vi "XImc example calb corr.vi"() -> ()   [LabVIEW 2012]
uses:
  libximc.lvlib
panel:
  in  "Correction table file.":path
  out "function return":i32
  out "Corrected position  Position":dbl
  out "Unrecorded position.":dbl
  in  "error in (no error)":errorcluster
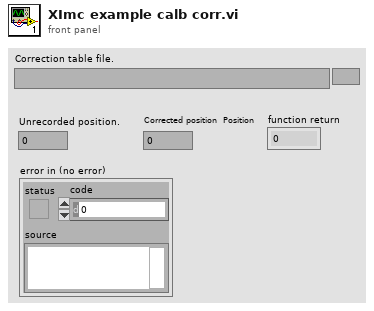
[diagram p1: front panel]
types:
  T1 = cluster{"NomVoltage":u32, "NomCurrent":u32, "NomSpeed":u32, "uNomSpeed":u32, "EngineFlags":u32, "Antiplay":i32, "MicrostepMode":u32, "StepsPerRev":u32}
  T2 = cluster{"Position":sgl, "@dummy control@":i8, "@dummy control@":i8, "@dummy control@":i8, "@dummy control@":i8, "EncPosition":i64}
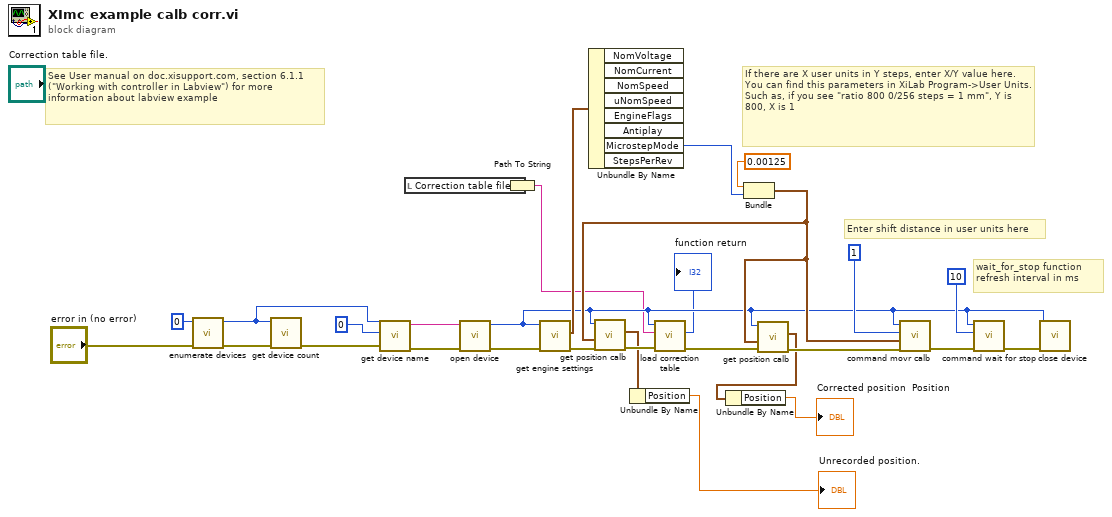
[diagram p0: block diagram]
diagram:
  # "See User manual on doc.xisupport.com, section 6.1.1 (\"Working with controller in Labview\") for more information about labview example"
  # "wait_for_stop function refresh interval in ms"
  # "Enter shift distance in user units here"
  # "If there are X user units in Y steps, enter X/Y value here.\nYou can find this parameters in XiLab Program->User Units.\nSuch as, if you see \"ratio 800 0/256 steps = 1 mm\", Y is 800, X is 1"
  n1 = call "enumerate devices.vi"("error in (no error)"="error in (no error)", "enumerate_flags"=0 ("probe_devices")) -> ("error out"=w27:errorcluster, "function return"=w25:u32)  [unwired: 8 in]
  n2 = call "get device count.vi"("error in (no error)"=w27, "device_enumeration"=w25) -> ("error out"=w26:errorcluster)  [unwired: 8 in, 1 out]
  n3 = call "get device name.vi"("error in (no error)"=w26, "device_index"=0 ("probe_devices"), "device_enumeration"=w25) -> ("error out"=w22:errorcluster, "function return"=w23:string)  [unwired: 7 in]
  n4 = local read "Correction table file."() -> (w2:path)
  n5 = call "open device.vi"("error in (no error)"=w22, "uri"=w23) -> ("error out"=w20:errorcluster, "function return"=w4:i32)  [unwired: 8 in]
  n6 = Path To String(path=w2) -> (string=w1:string)
  n7 = call "get engine settings.vi"("error in (no error)"=w20, "id"=w4) -> ("error out"=w13:errorcluster, "engine_settings out"=w19:T1)  [unwired: 7 in, 1 out]
  n8 = Unbundle By Name(w19) -> ("MicrostepMode"=w18:u32)  [unwired: 7 out]
  n9 = Bundle(0.00125, "MicrostepMode"=w18) -> (w11:cluster{dbl, "MicrostepMode":u32})  [unwired: 1 in]
  n10 = call "get position calb.vi"("error in (no error)"=w13, "calibration"=w11, "id"=w4) -> ("error out"=w12:errorcluster, "the_get_position_calb out"=w8:T2)  [unwired: 6 in, 1 out]
  n11 = Unbundle By Name(w8) -> ("Position"=→"Unrecorded position.":sgl)
  n12 = call "load correction table.vi"("error in (no error)"=w12, "namefile"=w1, "id"=w4) -> ("error out"=w10:errorcluster, "function return"=→"function return":i32)  [unwired: 6 in, 1 out]
  n13 = call "get position calb.vi"("error in (no error)"=w10, "calibration"=w11, "id"=w4) -> ("error out"=w9:errorcluster, "the_get_position_calb out"=w6:T2)  [unwired: 6 in, 1 out]
  n14 = Unbundle By Name(w6) -> ("Position"=→"Corrected position  Position":sgl)
  n15 = call "command movr calb.vi"("error in (no error)"=w9, "calibration"=w11, "DeltaPosition"=1 ("probe_devices"), "id"=w4) -> ("error out"=w16:errorcluster)  [unwired: 6 in, 1 out]
  n16 = call "command wait for stop.vi"("error in (no error)"=w16, "refresh_interval_ms"=10 ("probe_devices"), "id"=w4) -> ("error out"=w14:errorcluster)  [unwired: 7 in, 1 out]
  n17 = call "close device.vi"("error in (no error)"=w14, "id"=w4) -> ()  [unwired: 7 in, 3 out]
